vi "Configure Channels.vi"(8 "error in":errorcluster, 11 "AO DAQmx DC CFG in":refnum<class "AO DAQmx DC CFG.lvclass">) -> (0 "error out":errorcluster, 3 "AO DAQmx DC CFG out":refnum<class "AO DAQmx DC CFG.lvclass">)   [LabVIEW 2023, in "AO DAQmx DC CFG.lvclass"]
uses:
  AO DAQmx DC CFG.lvclass
  AO DAQmx DC CFG.lvclass/AO DAQmx DC CFG.ctl
  <vilib>/Utility/error.llb/Error Cluster From Error Code.vi
  <vilib>/ErrorRing/Error Ring.xnode
  DIO/DO DAQmx Fixed Freq PWM CFG/DO DAQmx Fixed Freq PWM CFG.lvclass
  2706bce0-41ed-4706-90a9-e9d573054dd0.vi
  Configuration/Configuration JSON/Configuration JSON Base/CFG JSON.lvclass
  DAQmx/DAQmx Base CFG/DAQmx Base CFG.lvclass
  <vilib>/DAQmx/create/channels.llb/DAQmx Create Channel (AO-Voltage-Basic).vi
  D:/git/HAL/HAL GOOP4/DAQmx/DAQmx Base CFG/DAQmx Base CFG.lvclass
  D:/git/HAL/HAL GOOP4/CFG Target/CFG Target.lvclass
  D:/git/HAL/HAL GOOP4/Configuration/Configuration Semaphore/CFG Semaphore.lvclass
  D:/git/HAL/HAL GOOP4/Configuration/Configuration JSON/Configuration JSON Base/CFG JSON.lvclass
  D:/git/HAL/HAL GOOP4/Interfaces/IConfigure/IConfigure.lvclass
  D:/git/HAL/HAL GOOP4/AO/AO DAQmx DC CFG/AO DAQmx DC CFG.lvclass
  D:/git/HAL/HAL GOOP4/DIO/DO DAQmx Fixed Freq PWM CFG/DO DAQmx Fixed Freq PWM CFG.lvclass
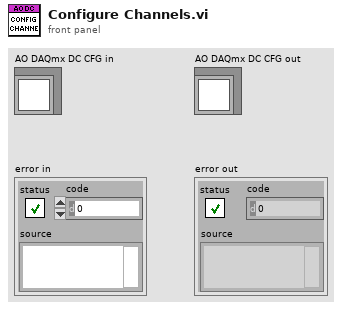
[diagram p1: front panel]
types:
  T1 = cluster{"Name":string, "Enabled":bool, "Maximum Value":dbl, "Minimum Value":dbl, "Output Terminal CFG":string, "Units":string}[]
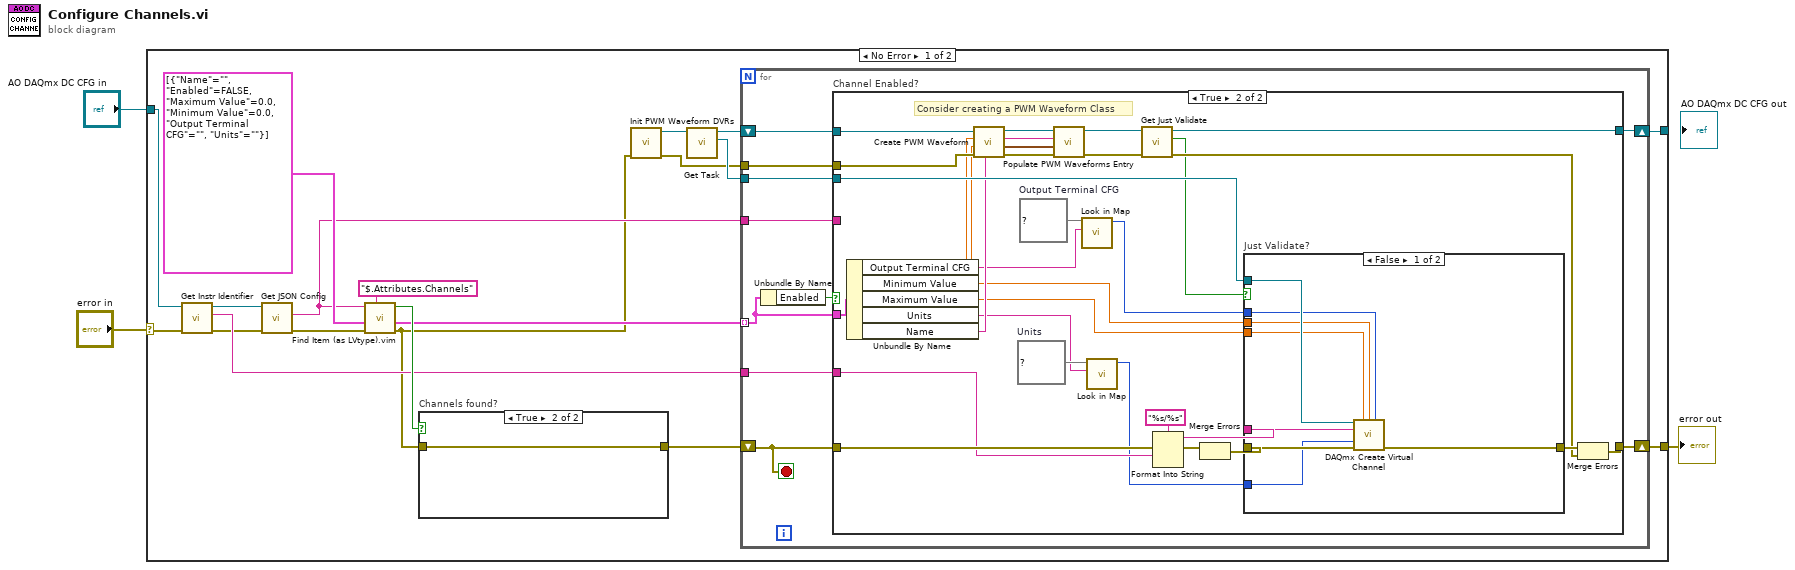
[diagram p0: block diagram]
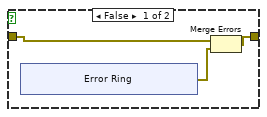
[diagram p2: hidden frame]
diagram:
  n1 = case shown="No Error" "error in" {
    selector: "error in" -> [w15 w81]
    tunnel: "AO DAQmx DC CFG in" -> [w11 w82]
    tunnel: [w16 w81] -> w1
    tunnel: [w10 w82] -> _
    frame No Error {
      n2 = call-dynamic "Get Instr Identifier.vi"("error in (no error)"=w15, "Configuration Base in"=w11) -> ("error out"=w4:errorcluster, "Instr Ident"=w17:string, "Configuration Base out"=w18:refnum<class "AO DAQmx DC CFG.lvclass">)  [unwired: 7 in]
      n3 = call "Get JSON Config.vi"("CFG Base in"=w18) -> ("<JSON>Config>"=w14:string)  [unwired: 9 in, 1 out]
      n4 = call "Find Item (as LVtype).vim"("$Path or Item Name"="$.Attributes.Channels", "error in (no error)"=w4, "Data Type and Default Value"=T1 [{"Name"="", "Enabled"=FALSE, "Maximum Value"=0.0, "Minimum Value"=0.0, "Output Terminal CFG"="", "Units"=""}], "JSON"=w14) -> ("error out"=w6:errorcluster, "Data"=w12:T1, "Found"=w20:bool)  [unwired: 4 in, 1 out]
      n5 = case "Channels found?" shown="True" w20 {
        tunnel: w6 -> [w24 w30]
        tunnel: [w22 w30] -> w8
        frame False {
          n6 = xnode "Error Ring"() -> ("error out"=w23:errorcluster)
          n7 = Merge Errors(w24, w23) -> (w22:errorcluster)
        }
        frame True {
        }
      }
      n8 = call "Init PWM Waveform DVRs.vi"("error in"=w6) -> ("error out"=w5:errorcluster, "DO DAQmx Fixed Freq PWM CFG out"=w7:refnum<class "DO DAQmx Fixed Freq PWM CFG.lvclass">)  [unwired: 9 in]
      n9 = call "Get Task.vi"("DAQmx Base CFG in"=w7) -> ("Task"=w13:refnum<k21>, "DAQmx Base CFG out"=w9:refnum<class "DO DAQmx Fixed Freq PWM CFG.lvclass">)  [unwired: 9 in]
      n10 = for {
        tunnel: w12 -> [w37] mode=indexing
        shift-right: [w40] -> w16
        shift-left: w8 -> [w39]
        tunnel: w17 -> [w38]
        tunnel: w14 -> [w36]
        tunnel: w13 -> [w35]
        shift-right: [w34] -> w10
        shift-left: w9 -> [w33]
        tunnel: w5 -> [w32]
        stop <- w39 stop-if-true
        n11 = Unbundle By Name(w37) -> ("Enabled"=w31:bool)
        n12 = case "Channel Enabled?" shown="True" w31 {
          tunnel: [w42 w69] -> w40
          tunnel: w39 -> [w42 w64]
          tunnel: w38 -> [_ w63]
          tunnel: w37 -> [_ w71]
          tunnel: [w41 w49] -> w34
          tunnel: w36 -> [_ _]
          tunnel: w35 -> [_ w67]
          tunnel: w33 -> [w41 w66]
          tunnel: w32 -> [_ w56]
          frame False {
          }
          frame True {
            w45 = map{string, i32} {"From Custom Scale"=10065, "Volts"=10348}  # Units
            w52 = map{string, i32} {"Default"=-1, "Differential"=10106, "Pseudodifferential"=12529, "RSE"=10083}  # Output Terminal CFG
            # "Consider creating a PWM Waveform Class"
            n13 = Unbundle By Name(w71) -> ("Output Terminal CFG"=w51:string, "Minimum Value"=w47:dbl, "Maximum Value"=w46:dbl, "Units"=w44:string, "Name"=w58:string)
            n14 = call-dynamic "Create PWM Waveform.vi"("Channel Ident"=w58, "error in"=w56, "Duty Cycle"=w46, "Frequency"=w47, "DO DAQmx Fixed Freq PWM CFG in"=w66) -> ("error out"=w60:errorcluster, "PWM Waveform"=w54:digitalwaveform, "Channel Ident out"=w55:string, "DO DAQmx Fixed Freq PWM CFG out"=w59:refnum<class "DO DAQmx Fixed Freq PWM CFG.lvclass">)  [unwired: 3 in]
            n15 = call "Populate PWM Waveforms Entry.vi"("error in"=w60, "PWM Waveform"=w54, "Channel Ident"=w55, "DO DAQmx Fixed Freq PWM CFG in"=w59) -> ("error out"=w68:errorcluster, "DO DAQmx Fixed Freq PWM CFG in 2"=w53:refnum<class "DO DAQmx Fixed Freq PWM CFG.lvclass">)  [unwired: 6 in]
            n16 = call "Look in Map.vi"("Key"=w51, "Map"=w52) -> ("Value"=w50:i32)  [unwired: 8 in, 1 out]
            n17 = call "Look in Map.vi"("Key"=w44, "Map"=w45) -> ("Value"=w43:i32)  [unwired: 8 in, 1 out]
            n18 = call "Get Just Validate.vi"("CFG JSON Base in"=w53) -> ("Just Validate"=w48:bool, "CFG JSON Base out"=w49:refnum<class "DO DAQmx Fixed Freq PWM CFG.lvclass">)  [unwired: 9 in]
            n19 = Format Into String(format string="%s/%s", error in=w64, w63) -> (resulting string=w61:string, error out=w62:errorcluster)  [unwired: 2 in]
            n20 = Merge Errors(w62) -> (w57:errorcluster)  [unwired: 1 in]
            n21 = case "Just Validate?" shown="False" w48 {
              tunnel: w57 -> [w79 w80]
              tunnel: w61 -> [w76 _]
              tunnel: w67 -> [w78 _]
              tunnel: [w77 w80] -> w70
              tunnel: w50 -> [w75 _]
              tunnel: w47 -> [w74 _]
              tunnel: w46 -> [w73 _]
              tunnel: w43 -> [w72 _]
              frame False {
                n22 = call-poly <vilib>:"DAQmx Create Virtual Channel.vi"("task in"=w78, "maximum value"=w73, "minimum value"=w74, "output terminal configuration"=w75, "physical channels"=w76, "units"=w72, "error in"=w79) -> ("error out"=w77:errorcluster)  [unwired: 7 in, 1 out]
              }
              frame True {
              }
            }
            n23 = Merge Errors(w70, w68) -> (w69:errorcluster)
          }
        }
      }
    }
    frame Error {
    }
  }
  "error out" <- w1
